vi "MessageName.vi"() -> (2 "MessageName":string)   [LabVIEW 2020, in "Event.lvlib"]
uses:
  Event.lvlib
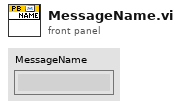
[diagram p1: front panel]
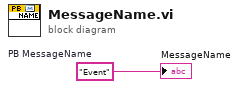
[diagram p0: block diagram]
diagram:
  w1 = "Event"  # PB MessageName
  "MessageName" <- w1
